vi "Pike Loop.vi"() -> ()   [LabVIEW 2014]
uses:
  Pike State.ctl
  Robot Code/Robot Global Data.vi
  Pike Mode.ctl
  Pike Command.ctl
panel:
  in  "Pike Command":T1
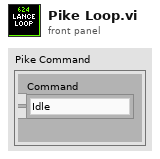
[diagram p1: front panel]
types:
  T1 = typedef "Pike Command.ctl" = cluster{"Command":T2}
  T2 = typedef "Pike Mode.ctl" = enum16{"Idle", "Auto Down", "Auto Up", "Manual Down", "Manual Up"}
  T3 = typedef "Pike State.ctl" = enum16{"Up", "Down", "Going Up", "Going Down"}
  T4 = typedef "Dashboard Control Data.ctl" = cluster{"Cam Exposure":dbl, "Go to angle":dbl, "Steer PID Gains":cluster{"proportional gain (Kc)":dbl, "integral time (Ti, min)":dbl, "derivative time (Td, min)":dbl}, "Steer PID output Range":cluster{"output high":dbl, "output low":dbl}, "Pressure m \nValue":dbl, "Pressure b \nValue":dbl, "Roller Command Cluster ":T5, "Elevator":T6, "Encoder Control":T8, "Auton Settings":cluster{"Drive Dist Window Size":dbl}, "Drivetrain Settings":T9, "Lance":T10}
  T5 = typedef "Roller Control.ctl" = cluster{"Intake Speed":dbl, "Turn In Speed":dbl, "Unload Speed":dbl, "Turn Out Speed":dbl, "Ping Align Tolerance":dbl, "Tote Range Threshold":dbl, "Right Pot 0":dbl, "Pot Threshold":dbl, "Left Pot 0":dbl, "Manual 0s?":bool, "Right Pot Scale":dbl, "Left Pot Scale":dbl, "0 wait time":i32, "Zero Pots":bool, "Min Elevator Height":dbl, "Eject Time":dbl, "Eject US Threshold":dbl, "Anti-Twitch Time":u32, "Ping Caring Threshold":dbl, "Pot Diff Threshold":dbl, "Pinch Sustain":u32, "Absorb Give Up Threshold":dbl, "Untip In Threshold":dbl, "Untip Grab Range":dbl, "Ultrasonic Hold Time":u32, "Landscape Absorb Time":u32, "Pot Use Wait Time":u32, "Can Turn Stop Range":dbl, "Ignore Pressure":bool, "HP Load Speed":dbl}
  T6 = typedef "Elevator DB Control.ctl" = cluster{"PID Output Range":cluster{"output high":dbl, "output low":dbl}, "PID gains":cluster{"proportional gain (Kc)":dbl, "integral time (Ti, min)":dbl, "derivative time (Td, min)":dbl}, "Height Tolerance":sgl, " Encoder Constant":dbl, "Safe Mode Max Speed":sgl, "Eject Time":sgl, "Zeroing Speed":sgl, "Presets":T7, "Ping Detect Threshold":sgl, "Trashcan Detect Threshold":sgl, "Zero Filter Time":dbl, "Stabilizer Open Time":dbl, "Zero Creep Speed":dbl, "Max Current":dbl, "Current Trip Time":dbl, "Abort Pitch":dbl, "Finger m":dbl, "Finger b":dbl, "Finger max ":dbl, "Finger Stabilizer":dbl, "Finger Store":dbl, "Finger Stop Store":dbl, "Stabilizer Close Time":dbl, "HP Finger Store":dbl, "HP Finger Stop Store":dbl, "Finger min":dbl, "Unstick gain":dbl, "Roller Wait":dbl}
  T7 = typedef "Elevator Presets.ctl" = cluster{"Pickup 2 w/ Tote":sgl, "Pickup 2 w/ Trashcan":sgl, "Pickup 3 w/ Tote":sgl, "Pickup 3 w/ Trashcan":sgl, "Bottom":sgl, "Pickup 1 w/ Tote":sgl, "Pickup Trashcan":sgl, "Pickup 1 w/ Trashcan":sgl, "Eject":sgl, "Hold Low":sgl, "Step add height":sgl, "Untip Lift":dbl, "Drop Stack":dbl, "HP Load Hold":dbl, "HP Load Drop":dbl, "HP Load Finger":dbl, "HP Load Hold Can":dbl, "Store can max":dbl, "HP Drag Score":dbl, "HP Store can max":dbl, "HP Drag Finish":dbl, "HP Carry min":dbl, "HP Finger Anti-Crash":dbl, "Finger trashcan avoid":dbl}
  T8 = typedef "Encoder Control.ctl" = cluster{"Left Tick Constant":dbl, "Right Tick Constant":dbl, "Center Tick Constant":dbl, "Reset?":bool, "Y Dist":cluster{"PID gains":cluster{"proportional gain (Kc)":dbl, "integral time (Ti, min)":dbl, "derivative time (Td, min)":dbl}}, "X Dist":cluster{"PID gains":cluster{"proportional gain (Kc)":dbl, "integral time (Ti, min)":dbl, "derivative time (Td, min)":dbl}}, "Y Stop Thresh":dbl, "Y Stop Speed":dbl, "X Stop Thresh":dbl, "X Stop Speed":dbl}
  T9 = typedef "Drivetrain Settings.ctl" = cluster{"Gyro Tolerance":sgl, "Strafe Correct max steer":sgl, "Strafe Timer Wait":sgl, "Throttle Ramp (ms)":sgl, "Strafe Ramp (ms)":sgl, "Angular rate compensation":bool, "Throttle to Rate Scale":sgl, "Rate compensation gain":sgl, "Creep Steer":sgl, "Creep Throttle":sgl}
  T10 = typedef "Pike DB Controls.ctl" = cluster{"Down Speed":dbl, "Up Speed":dbl, "Max Down Time":dbl, "Max Up Time":dbl, "Current Limit":dbl}
  T11 = typedef "WPI_DigitalInputDevRef.ctl" = cluster{"DevStatus":errorcluster, "DIO Channel":T12, "Controller":T13}
  T12 = typedef "FPGA_DIOChannel.ctl" = enum8{"DIO 0", "DIO 1", "DIO 2", "DIO 3", "DIO 4", "DIO 5", "DIO 6", "DIO 7", "DIO 8", "DIO 9", "DIO MXP 0", "DIO MXP 1", "DIO MXP 2", "DIO MXP 3", "DIO MXP 4", "DIO MXP 5", "DIO MXP 6", "DIO MXP 7", "DIO MXP 8", "DIO MXP 9", "DIO MXP 10", "DIO MXP 11", "DIO MXP 12", "DIO MXP 13", "DIO MXP 14", "DIO MXP 15", "Invalid"}
  T13 = typedef "FPGA_TypedefDigitalModule.ctl" = enum16{"Controller 1"}
  T14 = typedef "WPI_MotorControlDeviceRef.ctl" = cluster{"DeviceStatus":errorcluster, "Type":T15, "PWM":cluster{"Controller":T13, "PWM Channel":T16, "DeadBand":T17}, "CAN":cluster{"Device Number":u8, "Control Mode":T18, "Semaphore":T19, "Max Vout":dbl, "TalonSRX Control Mode":T20}, "Invert":bool, "TransformRef":T21, "InvTransformRef":T21}
  T15 = typedef "WPI_MotorControlType.ctl" = enum16{"PWM", "CAN", "CANTalonSRX"}
  T16 = typedef "FPGA_DIOPWMChannel.ctl" = enum8{"PWM 0", "PWM 1", "PWM 2", "PWM 3", "PWM 4", "PWM 5", "PWM 6", "PWM 7", "PWM 8", "PWM 9", "PWM MXP 0", "PWM MXP 1", "PWM MXP 2", "PWM MXP 3", "PWM MXP 4", "PWM MXP 5", "PWM MXP 6", "PWM MXP 7", "PWM MXP 8", "PWM MXP 9", "Invalid"}
  T17 = typedef "WPI_PWMDeadband.ctl" = cluster{"Name":string, "maxPositivePwm":i32, "minPositivePwm":i32, "centerPwm":i32, "maxNegativePwm":i32, "minNegativePwm":i32, "angularRange":u16}
  T18 = typedef "WPI_CANJaguar_ControlMode.ctl" = enum8{"Percent VBus", "Current", "Speed", "Position", "Voltage"}
  T19 = typedef "Semaphore RefNum" = refnum<k1>
  T20 = typedef "WPI_CANTalonSRX_APIControlMode.ctl" = enum8{"Percent VBus", "Speed", "Position", "Slave", "Unchanged / Invalid"}
  T21 = typedef "WPI_PWMTransform_ConPane.ctl" = refnum<vi>
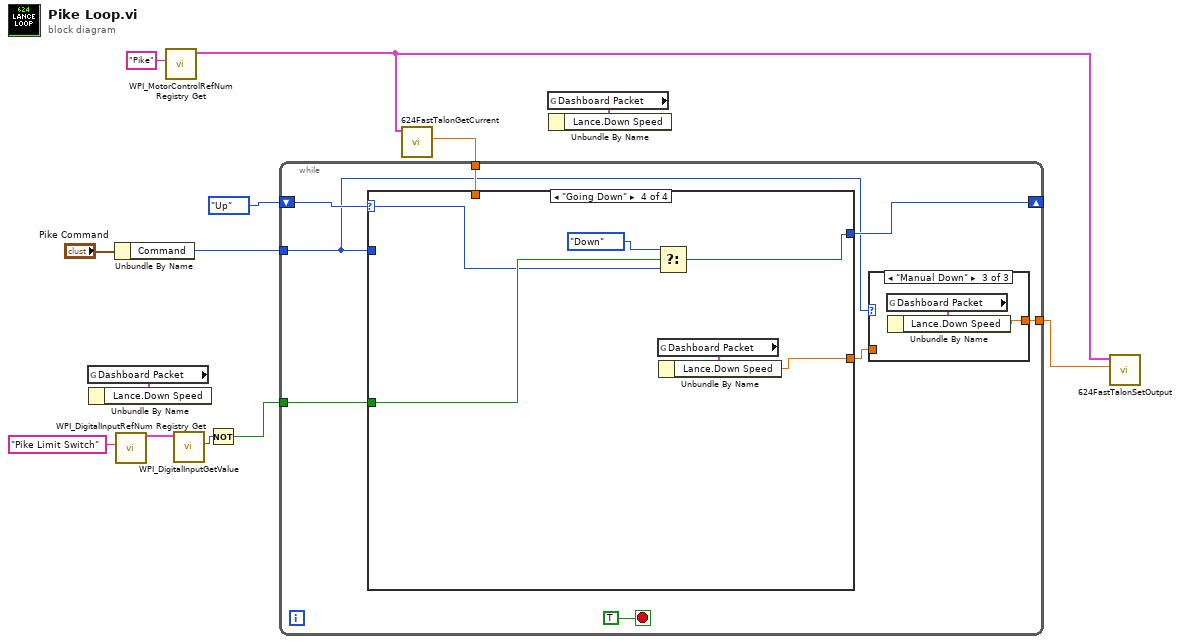
[diagram p0: block diagram]
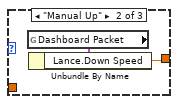
[diagram p3: hidden frame]
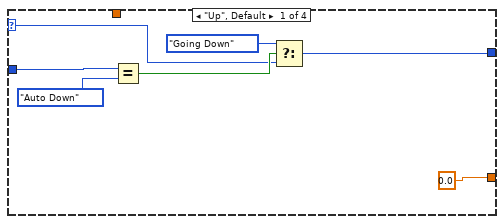
[diagram p4: hidden frame]
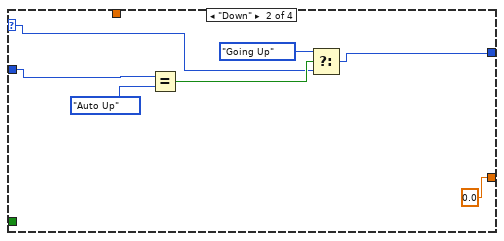
[diagram p5: hidden frame]
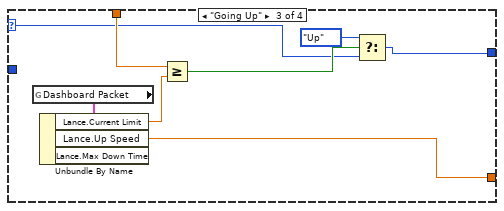
[diagram p6: hidden frame]
diagram:
  n1 = global read "Robot Global Data.vi" "Dashboard Packet"() -> (w11:T4)
  n2 = Unbundle By Name(w11) -> ()  [unwired: 1 out]
  n3 = Unbundle By Name("Pike Command") -> ("Command"=w8:T2)
  n4 = call <vilib>:"WPI_DigitalInputRefNum Registry Get.vi"("refnum name"="Pike Limit Switch") -> ("DigitalInputDevRef"=w4:T11)  [unwired: 9 in, 1 out]
  n5 = call <vilib>:"WPI_MotorControlRefNum Registry Get.vi"("refnum name"="Pike") -> ("MotorControlDevRef"=w7:T14)  [unwired: 9 in, 1 out]
  n6 = call <vilib>:"WPI_DigitalInputGetValue.vi"("DigitalInputDevRef"=w4) -> ("Value"=w3:bool)  [unwired: 8 in, 2 out]
  n7 = Not(x=w3) -> (.not. x?=w2:bool)
  n8 = call "624FastTalonGetCurrent.vi"("CAN Talon SRX Ref"=w7) -> ("Current"=w6:dbl)  [unwired: 10 in]
  n9 = while {
    shift-right: [w19] -> _
    shift-left: Pike_State."Up" -> [w20]
    tunnel: w8 -> [w16]
    tunnel: w6 -> [w18]
    tunnel: w2 -> [w17]
    tunnel: [w14] -> w1
    stop <- TRUE stop-if-true
    n10 = case shown="\"Going Down\"" w20 {
      selector: w20 -> [w29 w35 w43 w51]
      tunnel: [0.0 0.0 w46 w53] -> w15
      tunnel: w16 -> [w32 w36 _ _]
      tunnel: [w27 w34 w41 w49] -> w19
      tunnel: w18 -> [_ _ w47 _]
      tunnel: w17 -> [_ _ _ w52]
      frame "Up", Default {
        n11 = Equal?(x=w32, y=Pike_Mode."Auto Down") -> (x = y?=w30:bool)
        n12 = Select(t=Pike_State."Going Down", s=w30, f=w29) -> (s? t:f=w27:T3)
      }
      frame "Down" {
        n13 = Equal?(x=w36, y=Pike_Mode."Auto Up") -> (x = y?=w38:bool)
        n14 = Select(t=Pike_State."Going Up", s=w38, f=w35) -> (s? t:f=w34:T3)
      }
      frame "Going Up" {
        n15 = global read "Robot Global Data.vi" "Dashboard Packet"() -> (w48:T4)
        n16 = Unbundle By Name(w48) -> ("Lance.Current Limit"=w45:dbl, "Lance.Up Speed"=w46:dbl)  [unwired: 1 out]
        n17 = Greater Or Equal?(x=w47, y=w45) -> (x >= y?=w44:bool)
        n18 = Select(t=Pike_State."Up", s=w44, f=w43) -> (s? t:f=w41:T3)
      }
      frame "Going Down" {
        n19 = Select(t=Pike_State."Down", s=w52, f=w51) -> (s? t:f=w49:T3)
        n20 = global read "Robot Global Data.vi" "Dashboard Packet"() -> (w54:T4)
        n21 = Unbundle By Name(w54) -> ("Lance.Down Speed"=w53:dbl)
      }
    }
    n22 = case shown="\"Manual Down\"" w16 {
      tunnel: [w22 w23 w25] -> w14
      tunnel: w15 -> [w22 _ _]
      frame "Idle", Default {
      }
      frame "Manual Up" {
        n23 = global read "Robot Global Data.vi" "Dashboard Packet"() -> (w24:T4)
        n24 = Unbundle By Name(w24) -> ("Lance.Down Speed"=w23:dbl)
      }
      frame "Manual Down" {
        n25 = global read "Robot Global Data.vi" "Dashboard Packet"() -> (w26:T4)
        n26 = Unbundle By Name(w26) -> ("Lance.Down Speed"=w25:dbl)
      }
    }
  }
  n27 = global read "Robot Global Data.vi" "Dashboard Packet"() -> (w10:T4)
  n28 = Unbundle By Name(w10) -> ()  [unwired: 1 out]
  n29 = call "624FastTalonSetOutput.vi"("Output"=w1, "MotorControlDevRef"=w7) -> ()  [unwired: 8 in, 2 out]
